vi "PreCalc 2.0Frame Durations.vi"(8 "error in (no error)":errorcluster, 10 "Bit Time (seconds)":dbl, 11 "CANBus_Load_Calculator in":refnum<class "CANBus_Load_Calculator.lvclass">) -> (0 "error out":errorcluster, 3 "CANBus_Load_Calculator out":refnum<class "CANBus_Load_Calculator.lvclass">)   [LabVIEW 2019, in "XNET-Bus-Load-Calculator.lvlib" / "CANBus_Load_Calculator.lvclass"]
uses:
  CANBus_Load_Calculator.lvclass
  CANBus_Load_Calculator.lvclass/CANBus_Load_Calculator.ctl
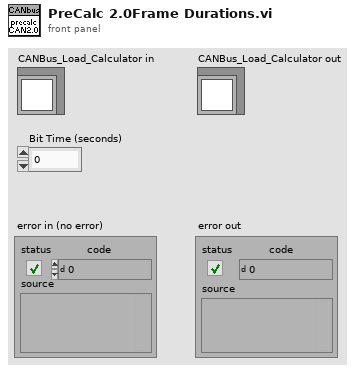
[diagram p1: front panel]
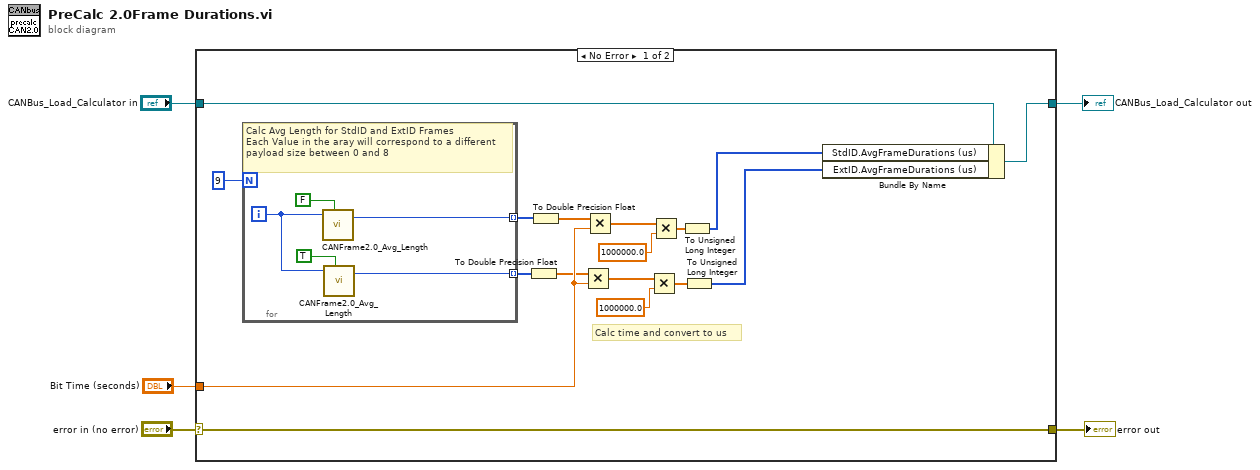
[diagram p0: block diagram]
diagram:
  n1 = case shown="No Error" "error in (no error)" {
    selector: "error in (no error)" -> [w6 w29]
    tunnel: "Bit Time (seconds)" -> [w21 _]
    tunnel: [w13 w28] -> w4
    tunnel: "CANBus_Load_Calculator in" -> [w12 w28]
    tunnel: [w6 w29] -> w1
    frame No Error {
      # "Calc time and convert to us"
      n2 = for {
        N: 9 -> [_]
        tunnel: [w26] -> w8 mode=indexing
        tunnel: [w23] -> w20 mode=indexing
        i -> [w24]
        # "Calc Avg Length for StdID and ExtID Frames\nEach Value in the aray will correspond to a different payload size between 0 and 8"
        n3 = call "CANFrame2.0_Avg_Length.vi"("Payload Size (bytes)"=w24, "Extended ID?"=FALSE) -> ("Avg.Length (bits)"=w26:i32)  [unwired: 4 in]
        n4 = call "CANFrame2.0_Avg_Length.vi"("Payload Size (bytes)"=w24, "Extended ID?"=TRUE) -> ("Avg.Length (bits)"=w23:i32)  [unwired: 4 in]
      }
      n5 = To Double Precision Float(number=w20) -> (double precision float=w16:dbl[])
      n6 = To Double Precision Float(number=w8) -> (double precision float=w9:dbl[])
      n7 = Multiply(x=w16, y=w21) -> (x*y=w17:dbl[])
      n8 = Multiply(x=w9, y=w21) -> (x*y=w10:dbl[])
      n9 = Multiply(x=w17, y=1000000.0) -> (x*y=w19:dbl[])
      n10 = Multiply(x=w10, y=1000000.0) -> (x*y=w14:dbl[])
      n11 = To Unsigned Long Integer(number=w14) -> (unsigned 32bit integer=w15:u32[])
      n12 = To Unsigned Long Integer(number=w19) -> (unsigned 32bit integer=w22:u32[])
      n13 = Bundle By Name(cluster=w12, "StdID.AvgFrameDurations (us)"=w15, "ExtID.AvgFrameDurations (us)"=w22) -> (w13:refnum<class "CANBus_Load_Calculator.lvclass">)
    }
    frame Error {
    }
  }
  "CANBus_Load_Calculator out" <- w4
  "error out" <- w1
